vi "sub_speaker_switch.vi"(8 "Active Speaker\n(Index)":i32=7, 9 "Num of Speakers":i32=7, 11 "task in":refnum<k21>="DigitalTest7") -> (0 "Array (Ausgang)":bool[](array[boolean]))   [LabVIEW 2014]
uses:
  <vilib>/DAQmx/write.llb/DAQmx Write (Digital 1D Bool NChan 1Samp 1Line).vi
panel:
  out "error out 2":errorcluster
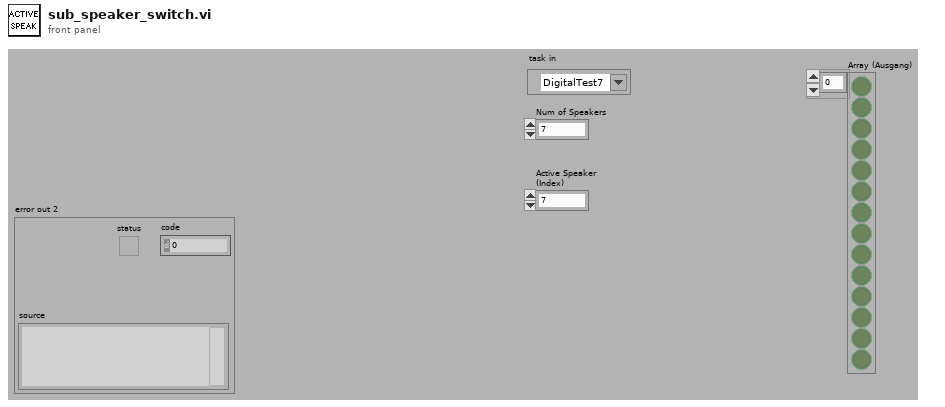
[diagram p1: front panel]
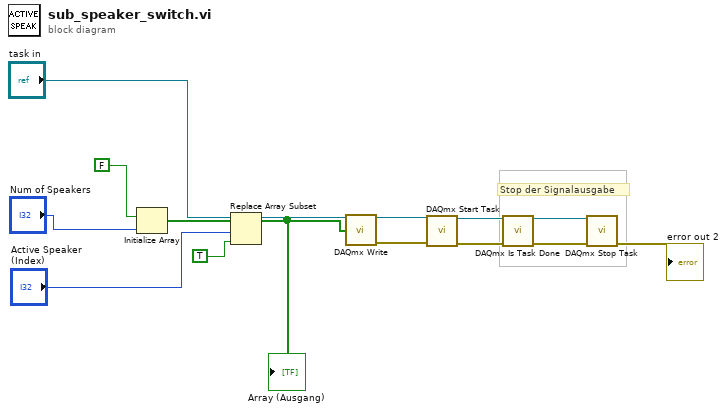
[diagram p0: block diagram]
diagram:
  # "Stop der Signalausgabe"
  n1 = Initialize Array(FALSE, "Num of Speakers") -> (w5:bool[])
  n2 = Replace Array Subset(array=w5, new element=TRUE, index="Active Speaker\n(Index)") -> (w2:bool[])
  "Array (Ausgang)" <- w2
  n3 = call-poly <vilib>:"DAQmx Write.vi"("task/channels in"="task in", "data"=w2) -> ("task out"=w14:refnum<k21>, "error out"=w13:errorcluster)  [unwired: 11 in, 1 out]
  n4 = call <vilib>:"DAQmx Start Task.vi"("task/channels in"=w14, "error in"=w13) -> ("task out"=w9:refnum<k21>, "error out"=w8:errorcluster)  [unwired: 12 in]
  n5 = call <vilib>:"DAQmx Is Task Done.vi"("task/channels in"=w9, "error in"=w8) -> ("task out"=w12:refnum<k21>, "error out"=w11:errorcluster)  [unwired: 11 in, 1 out]
  n6 = call <vilib>:"DAQmx Stop Task.vi"("task/channels in"=w12, "error in"=w11) -> ("error out"=→"error out 2":errorcluster)  [unwired: 12 in, 1 out]
